vi "MainHost.vi"() -> ()   [LabVIEW 2014]
panel:
  out "XY ActivePath":cluster{dbl[], dbl[]}(graph)
  out "e 2":dbl
  out "y2 2":dbl
  out "x2 2":dbl
  out "y1 2":dbl
  out "x1 2":dbl
  out "pathActive":string
  out "dpActive":string
  out "Heading":dbl
  out "Pos x":dbl
  out "Pos y":dbl
  in  "isHIL":bool
  out "alpha Saturated":bool
  out "u Saturated":bool
  out "u":dbl[](array[numeric])
  out "alpha":dbl[](array[numeric])
  out "?":picture
  out "Vessel position":cluster{"x":dbl[], "y":dbl[]}[](graph)
  in  "TabModes":T1(tab)
  in  "u thruster 1":dbl(slide) min=-1.0 max=1.0 scale=-1.0..1.0
  in  "alpha 1":dbl(knob) min=-114.0 max=114.0 scale=-114.0..114.0
  in  "u thruster 2":dbl(slide) min=-1.0 max=1.0 scale=-1.0..1.0
  in  "alpha 2":dbl(knob) min=-114.0 max=114.0 scale=-114.0..114.0
  in  "u thruster 0":dbl(slide) min=-1.0 max=1.0 scale=-1.0..1.0
  in  "alpha 0":dbl(knob) min=-114.0 max=114.0 scale=-114.0..114.0
  in  "Switch to dashboard control thrus":bool
  in  "Switch to dashboard control force":bool
  in  "N force":dbl step=0.1
  in  "Y force":dbl step=0.2
  in  "X force":dbl step=0.2
  out "Reference initialization completed":bool
  in  "PID gains psi":T2={"proportional gain (Kc)"=0.5, "integral time (Ti, min)"=0.0, "derivative time (Td, min)"=0.0}
  in  "PID gains y":T2={"proportional gain (Kc)"=0.5, "integral time (Ti, min)"=0.0, "derivative time (Td, min)"=0.0}
  in  "PID gains x":T2={"proportional gain (Kc)"=0.5, "integral time (Ti, min)"=0.0, "derivative time (Td, min)"=0.0}
  in  "psi dp":dbl
  in  "y dp":dbl
  in  "x dp":dbl
  in  "Activate DP":bool
  in  "TabPaths":enum32{"Straight line", "Ellipse", "Waypoints"}(tab)
  in  "u_r":dbl step=0.1
  in  "PID gains u straight":T2={"proportional gain (Kc)"=0.5, "integral time (Ti, min)"=0.0, "derivative time (Td, min)"=0.0}
  in  "Ok straight":bool
  in  "Clear straight":bool
  out "XY straight":cluster{"X":dbl, "Y":dbl}[](graph)
  in  "Preview ellipse":bool
  in  "e":dbl
  in  "y2":dbl
  in  "x2":dbl
  in  "y1":dbl
  in  "x1":dbl
  in  "Ok ellipse":bool
  in  "Clear ellipse":bool
  out "XY ellipse":cluster{"x":dbl[], "y":dbl[]}(graph)
  in  "Activate DP Mode":bool
  in  "Ok wp":bool
  in  "Clear wp":bool
  out "XY Waypoints":cluster{"X":dbl, "Y":dbl}[](graph)
  in  "stop":bool
  # "Starting procedure: Choose setpoint, gains and activate DP. \nThe vessel will respond when the reference model has finished initializing."
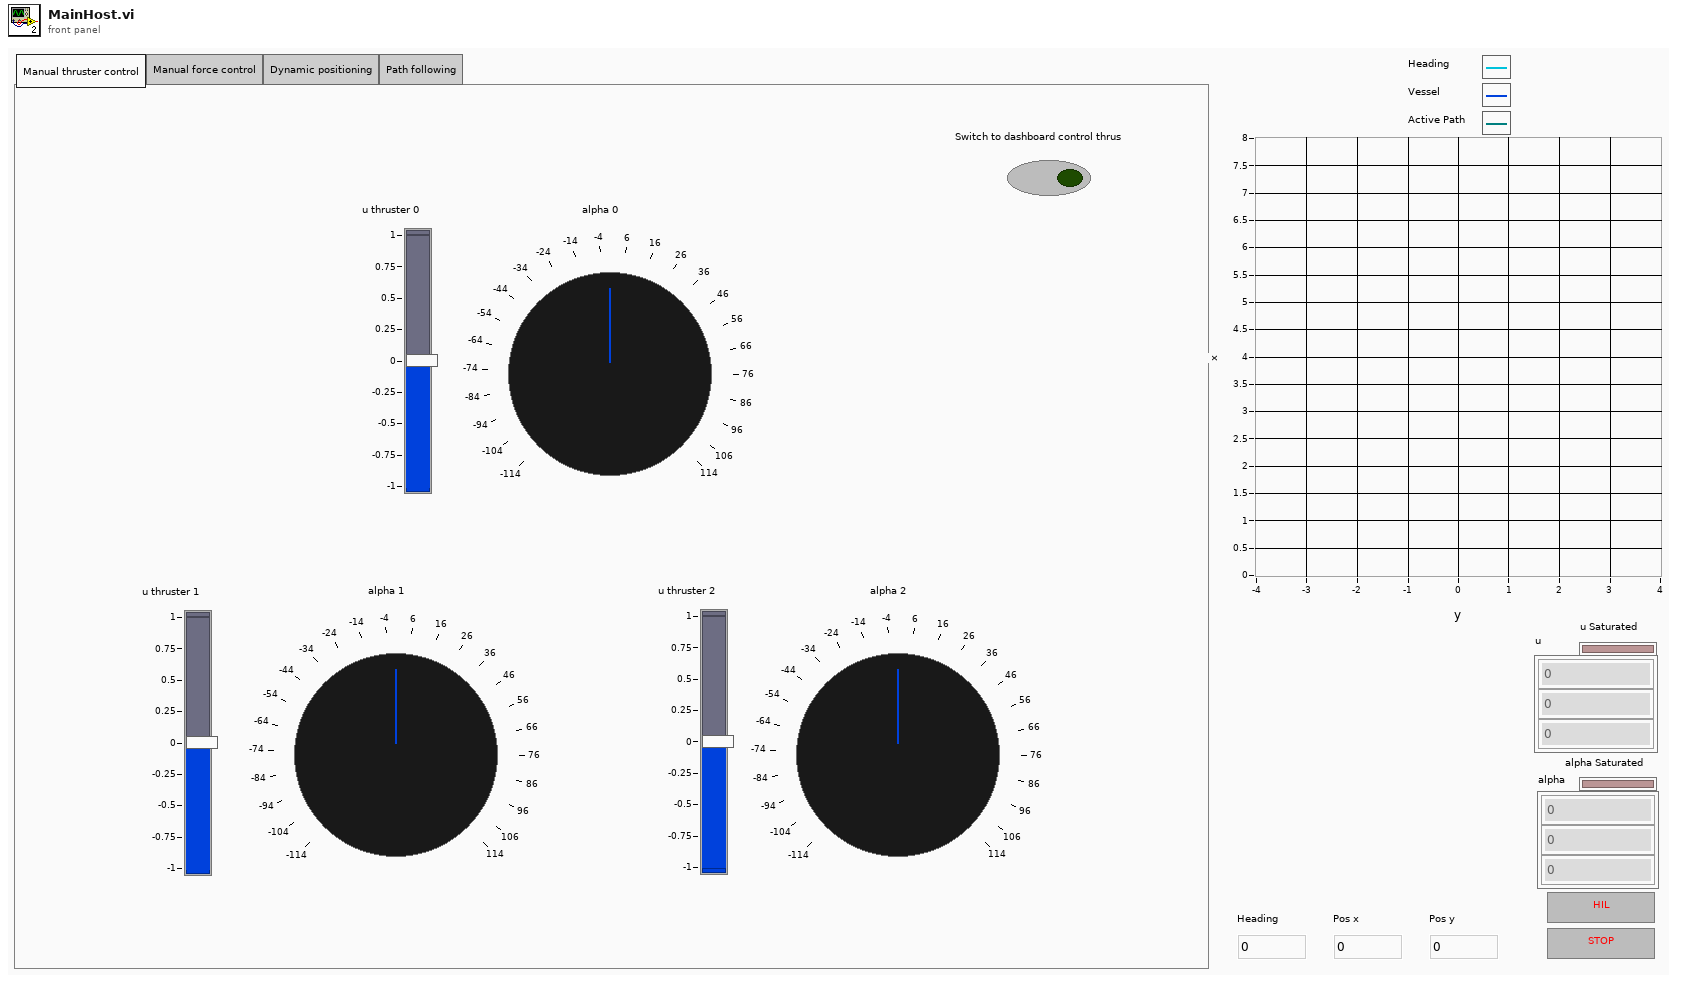
[diagram p1: front panel]
types:
  T1 = enum32{"Manual thruster control", "Manual force control", "Dynamic positioning", "Path following"}
  T2 = cluster{"proportional gain (Kc)":dbl, "integral time (Ti, min)":dbl, "derivative time (Td, min)":dbl}
  T3 = typedef "LVPoint32TypeDef.ctl" = cluster{"Horizontal":i32, "Vertical":i32}
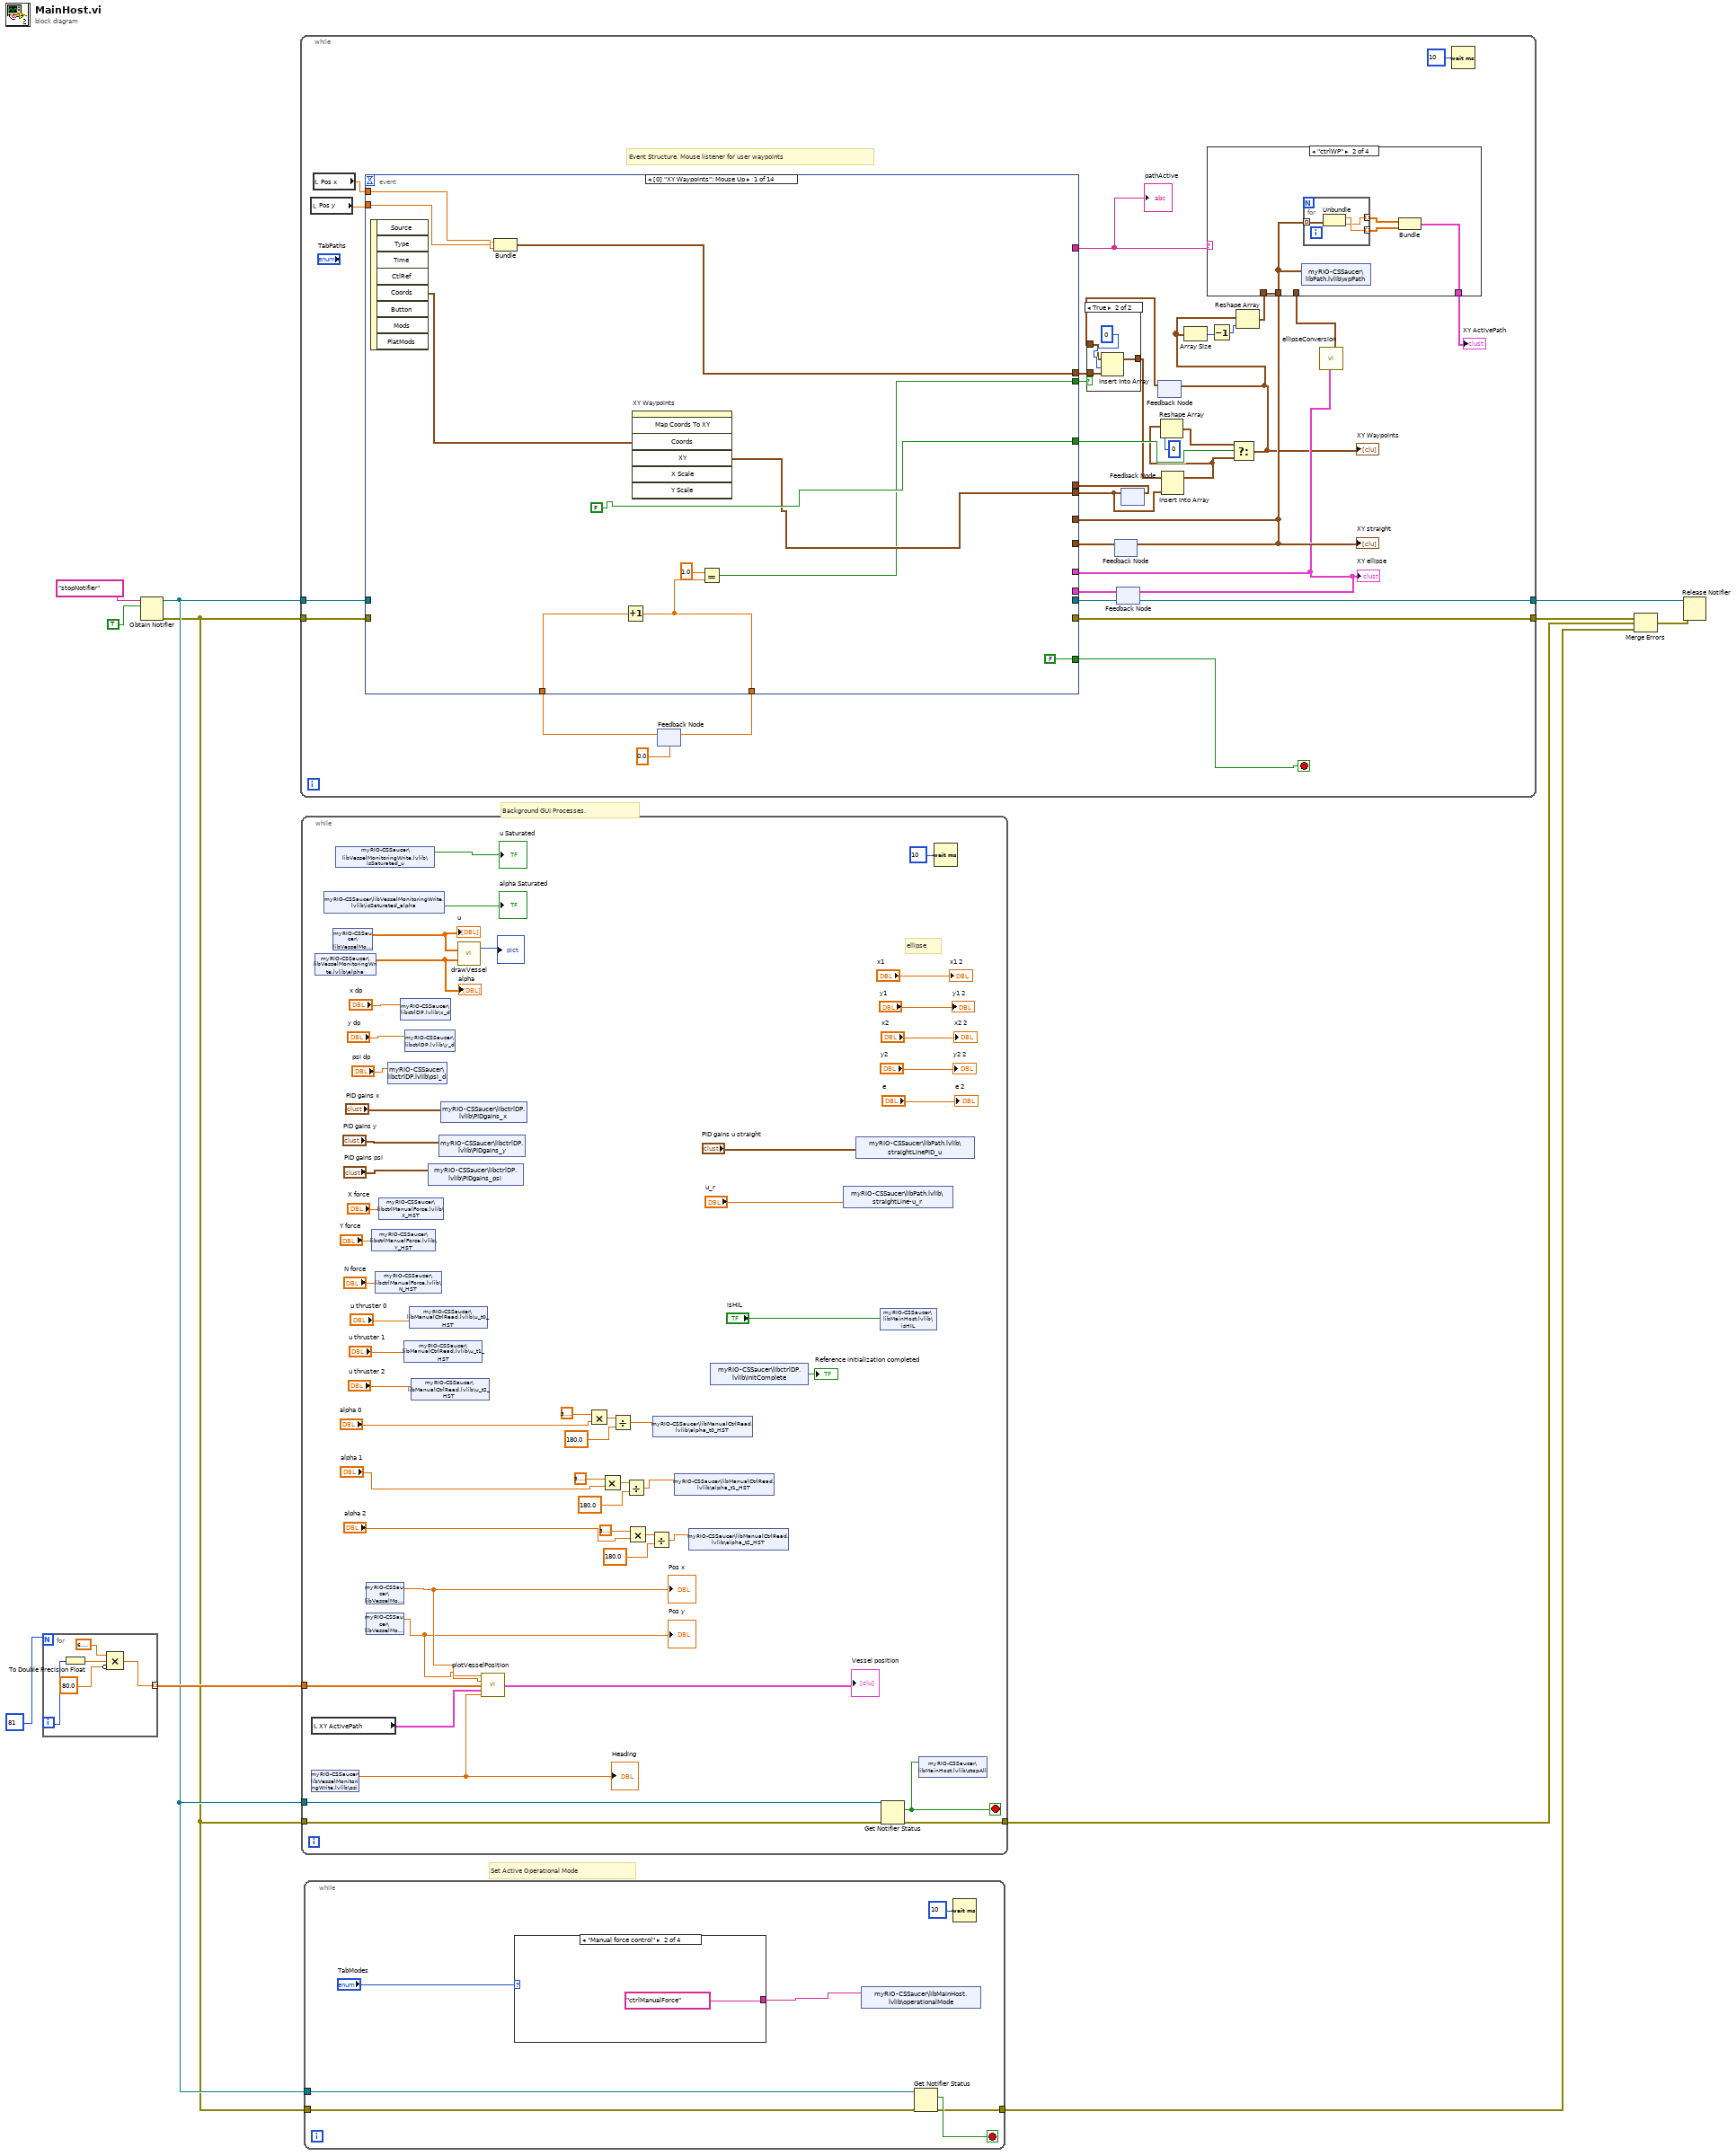
[diagram p0: block diagram]
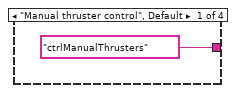
[diagram p2: hidden frame]
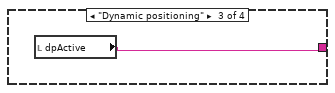
[diagram p3: hidden frame]
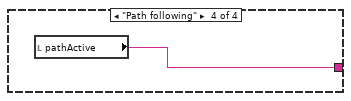
[diagram p4: hidden frame]
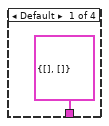
[diagram p6: hidden frame]
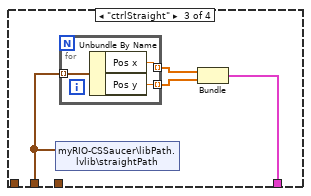
[diagram p7: hidden frame]
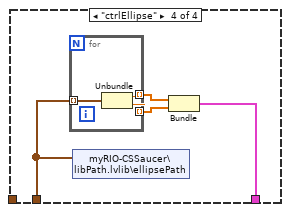
[diagram p8: hidden frame]
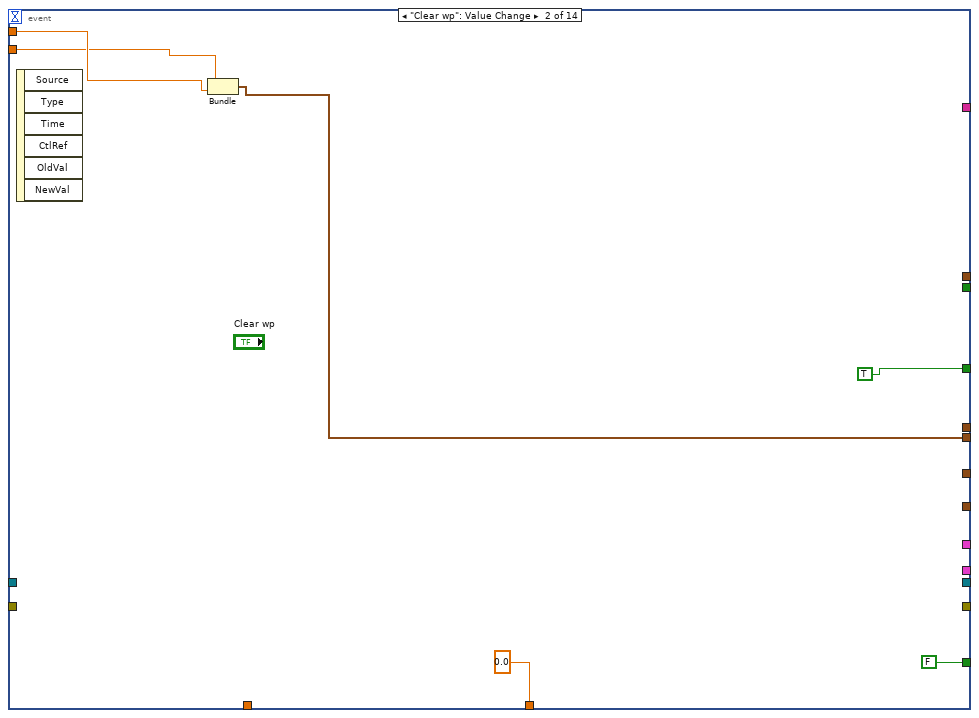
[diagram p9: hidden frame]
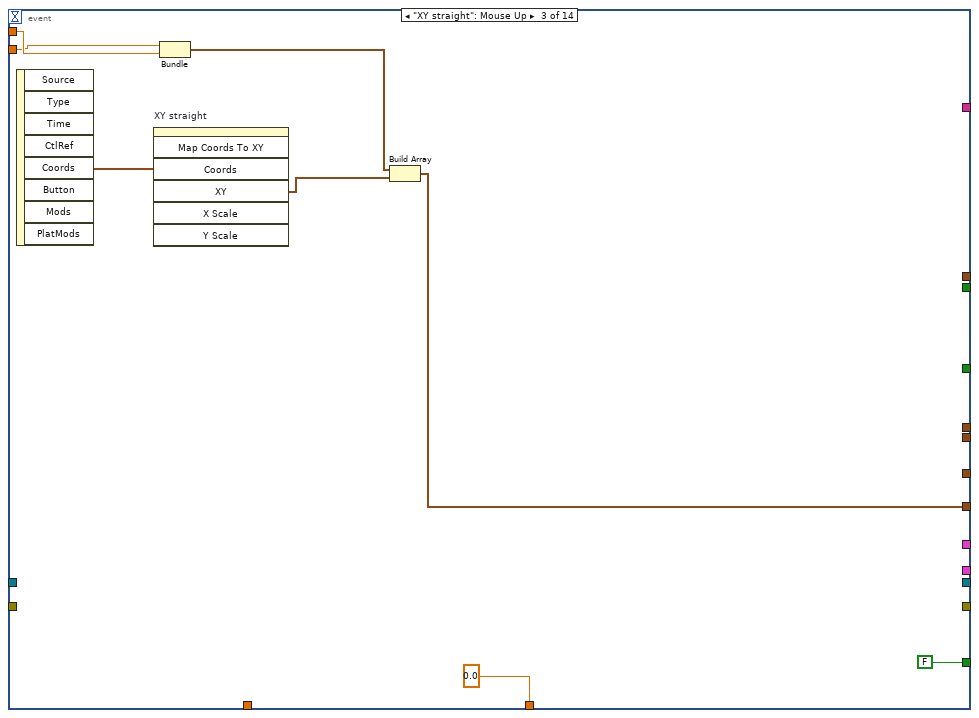
[diagram p10: hidden frame]
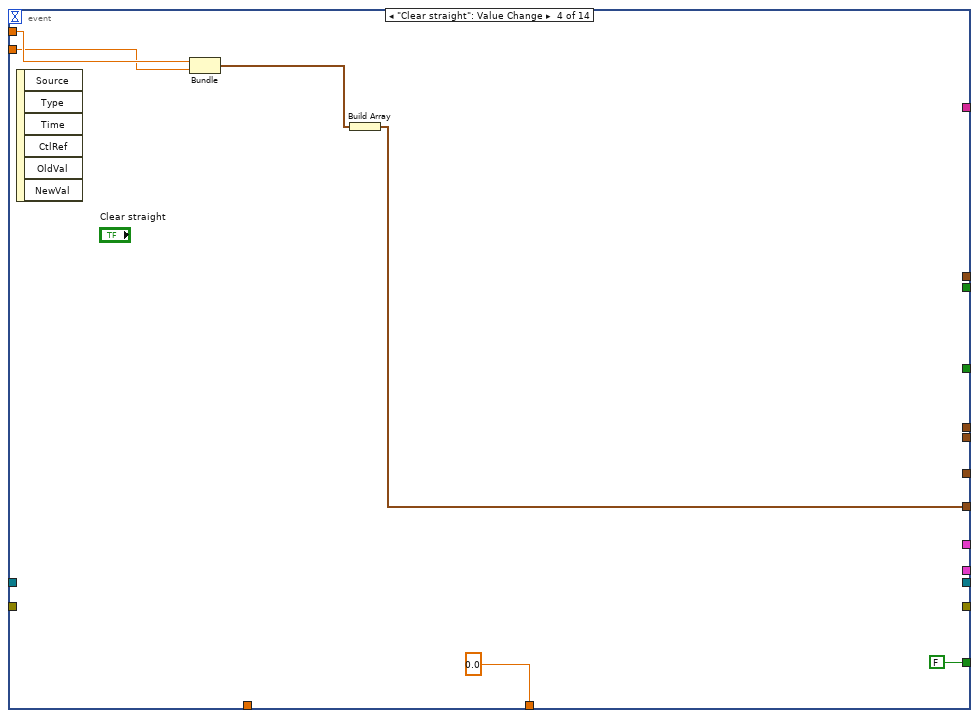
[diagram p11: hidden frame]
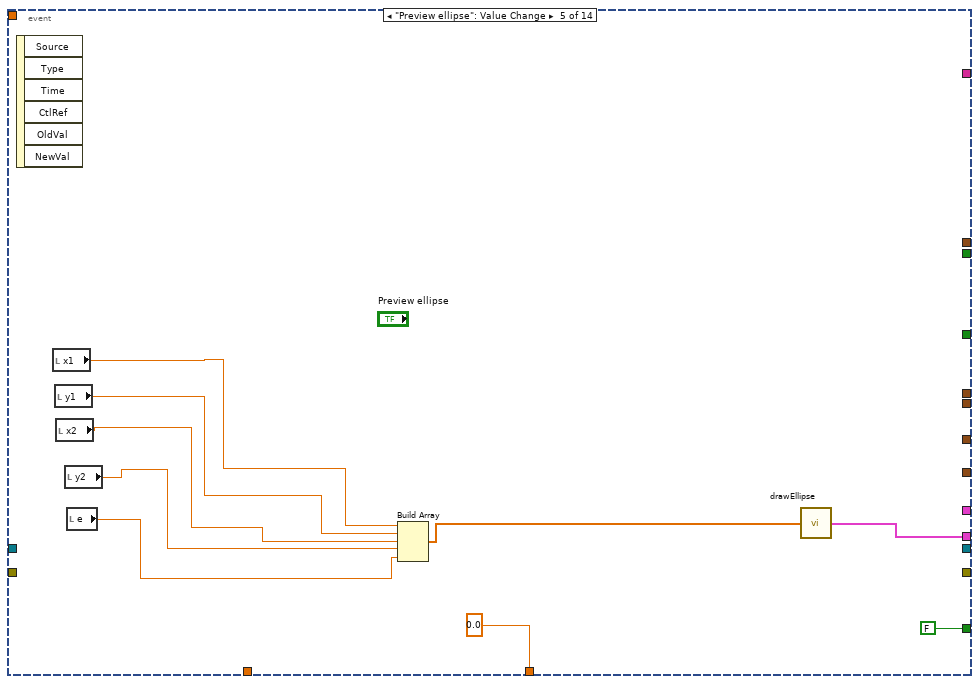
[diagram p12: hidden frame]
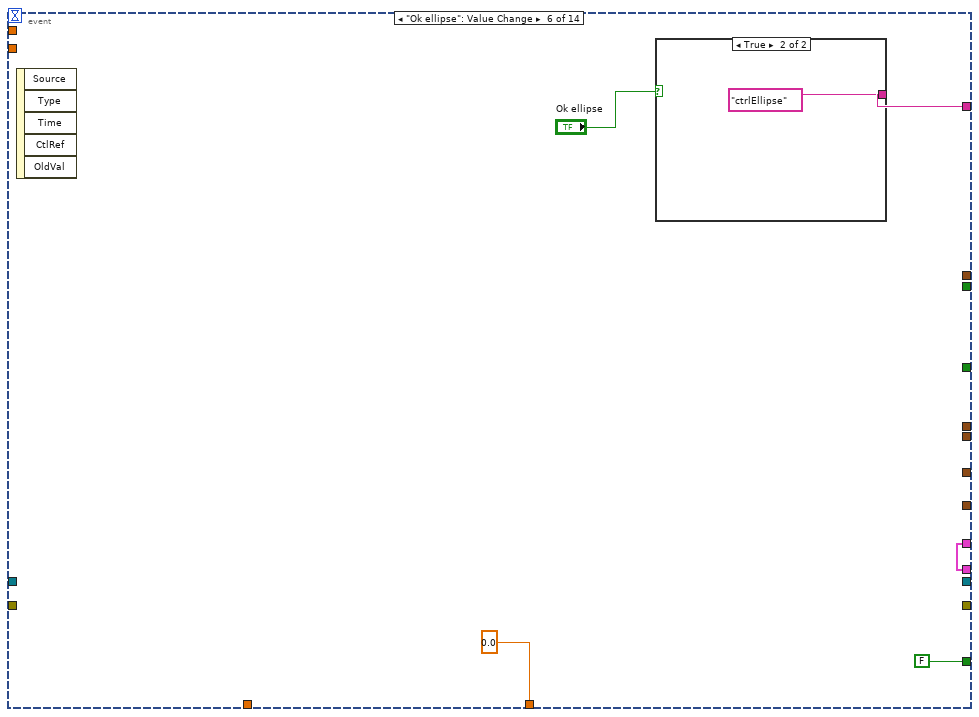
[diagram p13: hidden frame]
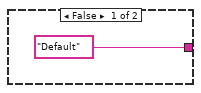
[diagram p14: hidden frame]
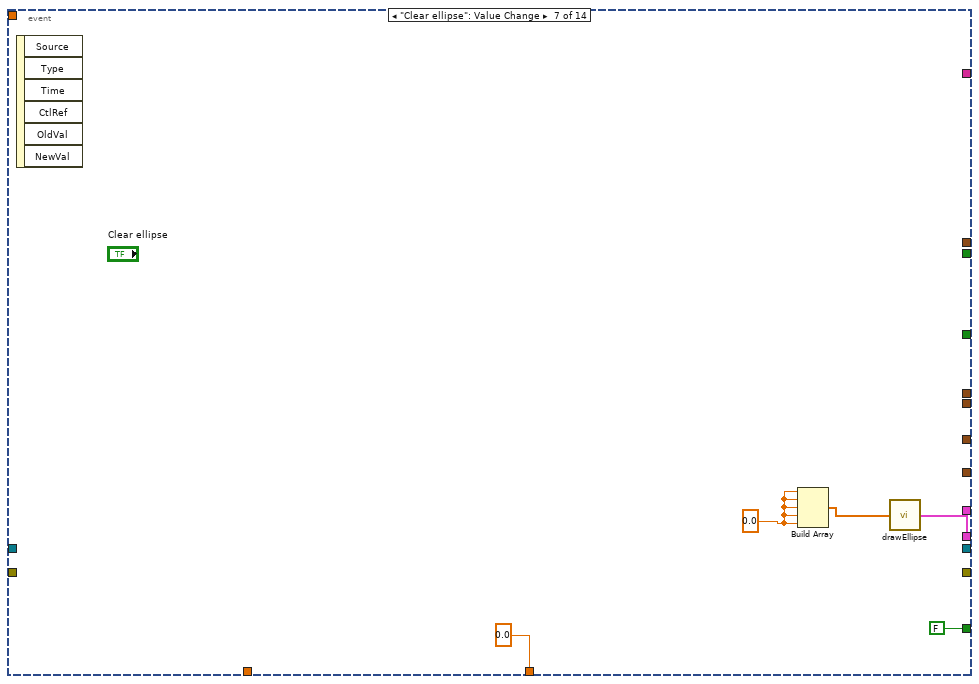
[diagram p15: hidden frame]
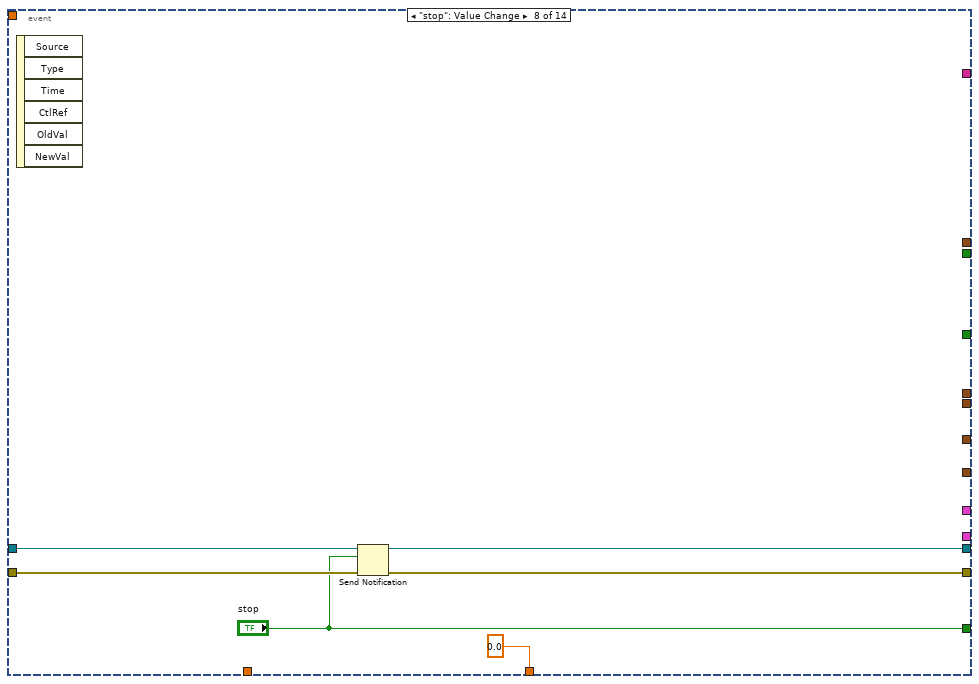
[diagram p16: hidden frame]
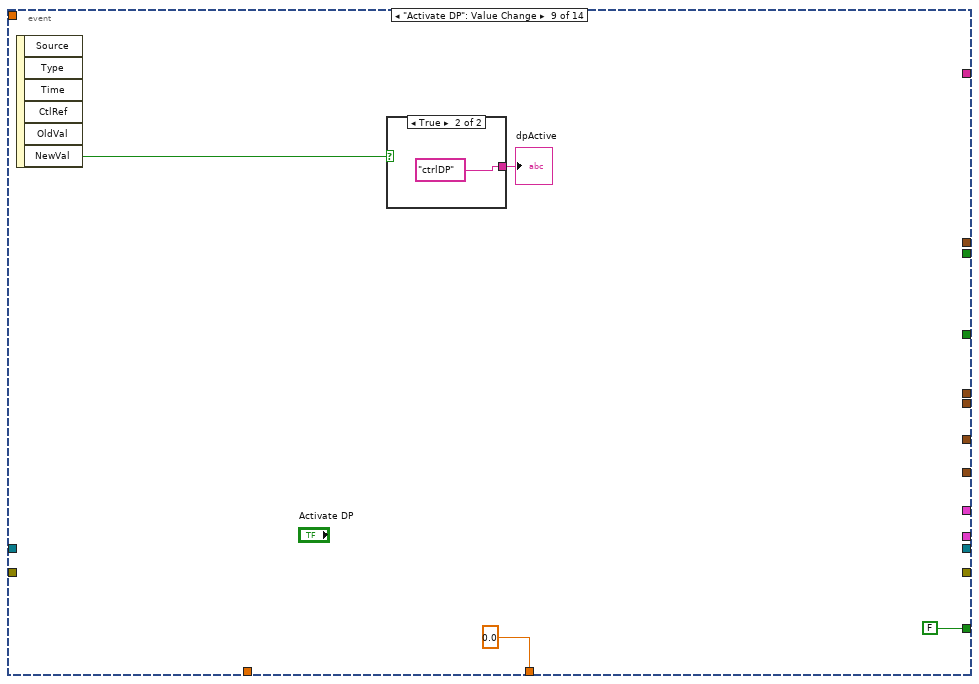
[diagram p17: hidden frame]
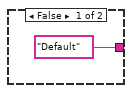
[diagram p18: hidden frame]
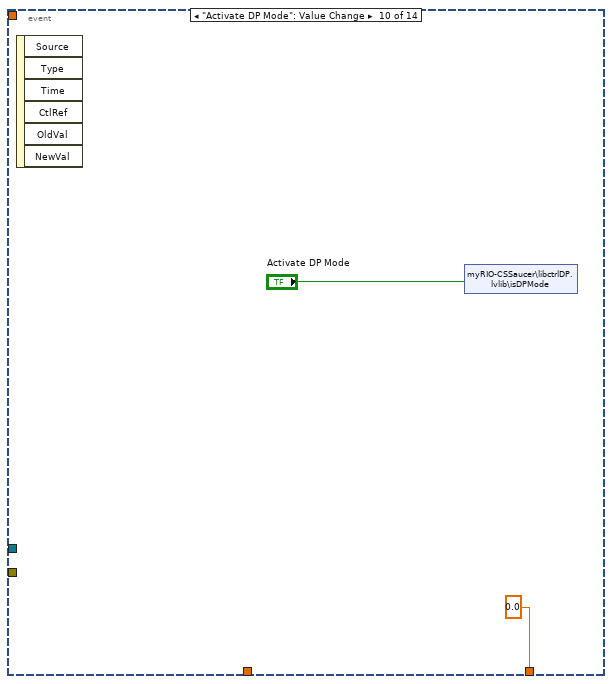
[diagram p19: hidden frame]
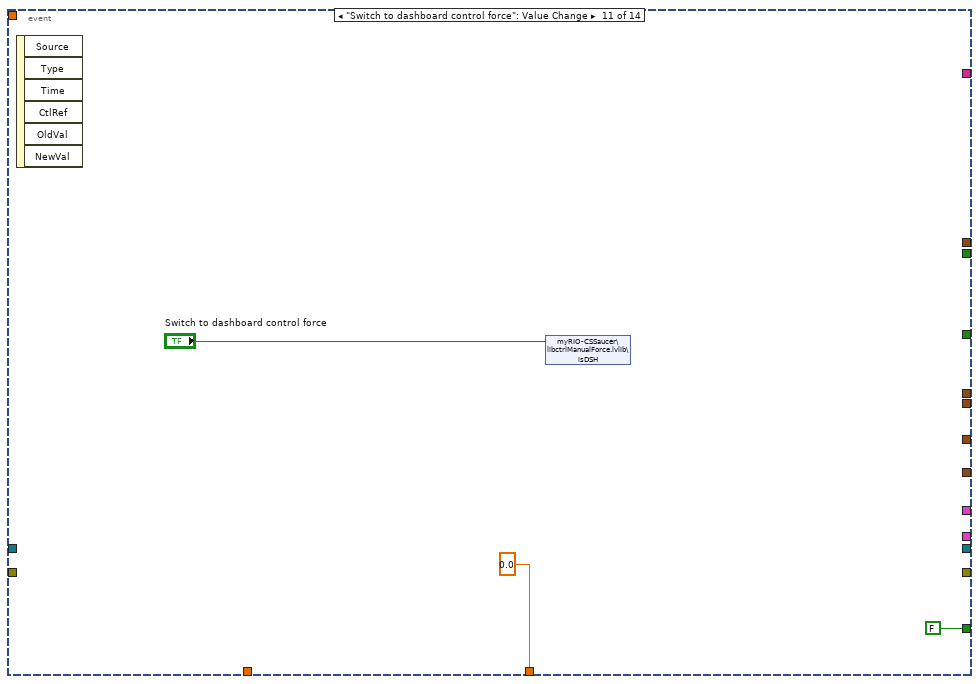
[diagram p20: hidden frame]
diagram:
  # "Background GUI Processes."
  # "Set Active Operational Mode"
  n1 = for {
    N: 81 -> [_]
    tunnel: [w12] -> w4 mode=indexing
    i -> [w14]
    n2 = To Double Precision Float(number=w14) -> (double precision float=w13:dbl)
    n3 = Compound Arithmetic op=MULTIPLY(6.283185307179586, w13, invert 80.0 ("value")) -> (w12:dbl)
  }
  n4 = Obtain Notifier(name (unnamed)="stopNotifier", notification data type=TRUE) -> (notifier out=w3:refnum<notifier>, error out=w2:errorcluster)  [unwired: 2 in, 1 out]
  n5 = while {
    tunnel: w3 -> [w43]
    tunnel: w2 -> [w42]
    tunnel: [w41] -> w7
    tunnel: [w40] -> w6
    stop <- w37 stop-if-true
    # "Event Structure. Mouse listener for user waypoints"
    n6 = local read "Pos y"() -> (w38:dbl)
    n7 = local read "Pos x"() -> (w39:dbl)
    n8 = feedback #1(0.0) -> (w21:dbl)
    n9 = feedback #2() -> (w34:cluster{"Pos x":dbl, "Pos y":dbl}[])  [unwired: 1 in]
    "XY straight" <- w34
    n10 = feedback #3() -> (w28:cluster{"x":dbl[], "y":dbl[]})  [unwired: 1 in]
    "XY ellipse" <- w28
    n11 = feedback #4() -> (w32:cluster{"Pos y":dbl, "Pos x":dbl})  [unwired: 1 in]
    n12 = event shown="[0] \"XY Waypoints\": Mouse Up" {
      selector: _ -> [_ _ _ _ _ _ _ _ _ _ _ _ _ _]
      dyn-events: _ -> [_ _ _ _ _ _ _ _ _ _ _ _ _ _]
      timeout: _ -> [_ _ _ _ _ _ _ _ _ _ _ _ _ _]
      tunnel: w38 -> [w76 w87 w93 w105 _ _ _ _ _ _ _ _ _ _]
      tunnel: w39 -> [w77 w88 w94 w106 _ _ _ _ _ _ _ _ _ _]
      tunnel: [_ _ w97 w103 _ _ _ _ _ _ _ _ w150 _] -> w35
      tunnel: [w84 w91 _ _ _ _ _ _ _ _ _ _ _ w155] -> w31
      tunnel: [FALSE TRUE _ _ _ _ _ _ _ _ _ _ _ _] -> w45
      tunnel: w43 -> [_ _ _ _ _ _ _ w133 _ _ _ _ _ _]
      tunnel: [_ _ _ _ _ _ _ w132 _ _ _ _ _ _] -> w41
      tunnel: w42 -> [_ _ _ _ _ _ _ w131 _ _ _ _ _ _]
      tunnel: [_ _ _ _ _ _ _ w130 _ _ _ _ _ _] -> w40
      tunnel: [FALSE FALSE FALSE FALSE FALSE FALSE FALSE "stop" FALSE _ FALSE FALSE FALSE FALSE] -> w37
      tunnel: [_ _ _ _ _ w120 _ _ _ _ _ _ w152 w158] -> w36
      tunnel: [_ _ _ _ w109 w118 w125 _ _ _ _ _ _ _] -> w33
      tunnel: w34 -> [_ _ _ _ _ _ _ _ _ _ _ _ w150 _]
      tunnel: w28 -> [_ _ _ _ _ w118 _ _ _ _ _ _ _ _]
      tunnel: w32 -> [_ _ _ _ _ _ _ _ _ _ _ _ _ w155]
      tunnel: w21 -> [w82 _ _ _ _ _ _ _ _ _ _ _ _ _]
      tunnel: [w81 0.0 0.0 0.0 0.0 0.0 0.0 0.0 0.0 0.0 0.0 0.0 0.0 _] -> w23
      tunnel: [w79 _ _ _ _ _ _ _ _ _ _ _ _ _] -> w18
      tunnel: [w78 _ _ _ _ _ _ _ _ _ _ _ _ _] -> w17
      event "XY Waypoints": Mouse Up {
        n13 = event-data() -> ("Coords"=w86:T3)  [unwired: 1 in, 7 out]
        n14 = Bundle("Pos y"=w76, "Pos x"=w77) -> (w79:cluster{"Pos y":dbl, "Pos x":dbl})  [unwired: 1 in]
        n15 = Increment(x=w82) -> (x+1=w81:dbl)
        n16 = invoke on="XY Waypoints" class="XYGraph (strict)" method="Map Coords To XY"("Coords"=w86) -> ("XY"=w84:cluster{"X":dbl, "Y":dbl})  [unwired: 6 in, 6 out]
        n17 = Equal?(x=1.0, y=w81) -> (x = y?=w78:bool)
      }
      event "Clear wp": Value Change {
        n18 = event-data() -> ()  [unwired: 1 in, 6 out]
        n19 = Bundle("Pos y"=w87, "Pos x"=w88) -> (w91:cluster{"Pos y":dbl, "Pos x":dbl})  [unwired: 1 in]
      }
      event "XY straight": Mouse Up {
        n20 = event-data() -> ("Coords"=w100:T3)  [unwired: 1 in, 7 out]
        n21 = invoke on="XY straight" class="XYGraph (strict)" method="Map Coords To XY"("Coords"=w100) -> ("XY"=w98:cluster{"X":dbl, "Y":dbl})  [unwired: 6 in, 6 out]
        n22 = Bundle("Pos y"=w93, "Pos x"=w94) -> (w99:cluster{"Pos y":dbl, "Pos x":dbl})  [unwired: 1 in]
        n23 = Build Array(w99, w98) -> (w97:cluster{"X":dbl, "Y":dbl}[])
      }
      event "Clear straight": Value Change {
        n24 = event-data() -> ()  [unwired: 1 in, 6 out]
        n25 = Bundle("Pos x"=w106, "Pos y"=w105) -> (w104:cluster{"Pos x":dbl, "Pos y":dbl})  [unwired: 1 in]
        n26 = Build Array(w104) -> (w103:cluster{"Pos x":dbl, "Pos y":dbl}[])
      }
      event "Preview ellipse": Value Change {
        n27 = event-data() -> ()  [unwired: 1 in, 6 out]
        n28 = local read "x1"() -> (w115:dbl)
        n29 = local read "y1"() -> (w114:dbl)
        n30 = local read "x2"() -> (w113:dbl)
        n31 = local read "y2"() -> (w112:dbl)
        n32 = local read "e"() -> (w111:dbl)
        n33 = Build Array(w115, w114, w113, w112, w111) -> (w110:dbl[])
        n34 = call "drawEllipse.vi"("ellipse in"=w110) -> ("XY ellipse"=w109:cluster{"x":dbl[], "y":dbl[]})  [unwired: 4 in]
      }
      event "Ok ellipse": Value Change {
        n35 = event-data() -> ()  [unwired: 1 in, 5 out]
        n36 = case shown="True" "Ok ellipse" {
          tunnel: ["Default" "ctrlEllipse"] -> w120
          frame False {
          }
          frame True {
          }
        }
      }
      event "Clear ellipse": Value Change {
        w127 = 0.0 ("element")
        n37 = event-data() -> ()  [unwired: 1 in, 6 out]
        n38 = Build Array(w127, w127, w127, w127, w127) -> (w126:dbl[])
        n39 = call "drawEllipse.vi"("ellipse in"=w126) -> ("XY ellipse"=w125:cluster{"x":dbl[], "y":dbl[]})  [unwired: 4 in]
      }
      event "stop": Value Change {
        n40 = event-data() -> ()  [unwired: 1 in, 6 out]
        n41 = Send Notification(notification="stop", notifier=w133, error in (no error)=w131) -> (notifier out=w132:refnum<notifier>, error out=w130:errorcluster)
      }
      event "Activate DP": Value Change {
        n42 = event-data() -> ("NewVal"=w137:bool)  [unwired: 1 in, 5 out]
        n43 = case shown="True" w137 {
          tunnel: ["Default" "ctrlDP"] -> w136
          frame False {
          }
          frame True {
          }
        }
        "dpActive" <- w136
      }
      event "Activate DP Mode": Value Change {
        n44 = event-data() -> ()  [unwired: 1 in, 6 out]
        n45 = shared-variable "myRIO-CSSaucer\\libctrlDP.lvlib\\isDPMode"("Activate DP Mode") -> ()  [unwired: 1 in, 1 out]
      }
      event "Switch to dashboard control force": Value Change {
        n46 = event-data() -> ()  [unwired: 1 in, 6 out]
        n47 = shared-variable "myRIO-CSSaucer\\libctrlManualForce.lvlib\\isDSH"("Switch to dashboard control force") -> ()  [unwired: 1 in, 1 out]
      }
      event "Switch to dashboard control thrus": Value Change {
        n48 = event-data() -> ()  [unwired: 1 in, 6 out]
        n49 = shared-variable "myRIO-CSSaucer\\libManualCtrlRead.lvlib\\isDashboardActive"("Switch to dashboard control thrus") -> ()  [unwired: 1 in, 1 out]
      }
      event "Ok straight": Value Change {
        n50 = event-data() -> ()  [unwired: 1 in, 6 out]
        n51 = case shown="True" "Ok straight" {
          tunnel: ["Default" "ctrlStraight"] -> w152
          frame False {
          }
          frame True {
          }
        }
      }
      event "Ok wp": Value Change {
        n52 = event-data() -> ()  [unwired: 1 in, 6 out]
        n53 = case shown="True" "Ok wp" {
          tunnel: ["Default" "ctrlWP"] -> w158
          frame False {
          }
          frame True {
          }
        }
      }
    }
    "pathActive" <- w36
    n54 = feedback-in #1(w23) -> ()
    n55 = feedback-in #2(w35) -> ()
    n56 = feedback-in #3(w33) -> ()
    n57 = feedback-in #4(w31) -> ()
    n58 = feedback #5() -> (w19:cluster{"Pos y":dbl, "Pos x":dbl}[])  [unwired: 1 in]
    n59 = case shown="True" w17 {
      tunnel: [w49 w50] -> w20
      tunnel: w19 -> [w49 w52]
      tunnel: w18 -> [_ w51]
      frame False {
      }
      frame True {
        n60 = Insert Into Array(array=w52, index=0, new element=w51) -> (w50:cluster{"Pos y":dbl, "Pos x":dbl}[])
      }
    }
    n61 = Insert Into Array(array=w20, new element=w31) -> (w44:cluster{"Pos y":dbl, "Pos x":dbl}[])  [unwired: 1 in]
    n62 = Reshape Array(w44, 0 ("dimension size")) -> (w47:cluster{"Pos y":dbl, "Pos x":dbl}[])
    n63 = Select(t=w47, s=w45, f=w44) -> (s? t:f=w26:cluster{"Pos y":dbl, "Pos x":dbl}[])
    "XY Waypoints" <- w26
    n64 = feedback-in #5(w26) -> ()
    n65 = Array Size(array=w26) -> (size(s)=w27:i32)
    n66 = Decrement(x=w27) -> (x-1=w25:i32)
    n67 = Reshape Array(w26, w25) -> (w24:cluster{"Pos y":dbl, "Pos x":dbl}[])
    n68 = call "ellipseConversion.vi"("XY ellipse 2"=w28) -> ("Array"=w30:cluster{dbl, dbl}[])  [unwired: 10 in]
    n69 = case shown="\"ctrlWP\"" w36 {
      tunnel: w34 -> [_ _ w65 _]
      tunnel: w24 -> [_ w58 _ _]
      tunnel: w30 -> [_ _ _ w72]
      tunnel: [cluster{dbl[], dbl[]} {[], []} w57 w64 w71] -> w29
      frame Default {
      }
      frame "ctrlWP" {
        n70 = shared-variable "myRIO-CSSaucer\\libPath.lvlib\\wpPath"(w58) -> ()  [unwired: 1 in, 1 out]
        n71 = for {
          tunnel: w58 -> [w61] mode=indexing
          tunnel: [w59] -> w56 mode=indexing
          tunnel: [w60] -> w55 mode=indexing
          n72 = Unbundle(w61) -> ("Pos y"=w60:dbl, "Pos x"=w59:dbl)
        }
        n73 = Bundle(w56, w55) -> (w57:cluster{dbl[], dbl[]})  [unwired: 1 in]
      }
      frame "ctrlStraight" {
        n74 = shared-variable "myRIO-CSSaucer\\libPath.lvlib\\straightPath"(w65) -> ()  [unwired: 1 in, 1 out]
        n75 = for {
          tunnel: w65 -> [w68] mode=indexing
          tunnel: [w67] -> w63 mode=indexing
          tunnel: [w66] -> w62 mode=indexing
          n76 = Unbundle By Name(w68) -> ("Pos x"=w67:dbl, "Pos y"=w66:dbl)
        }
        n77 = Bundle(w63, w62) -> (w64:cluster{dbl[], dbl[]})  [unwired: 1 in]
      }
      frame "ctrlEllipse" {
        n78 = for {
          tunnel: w72 -> [w75] mode=indexing
          tunnel: [w74] -> w69 mode=indexing
          tunnel: [w73] -> w70 mode=indexing
          n79 = Unbundle(w75) -> (w74:dbl, w73:dbl)
        }
        n80 = shared-variable "myRIO-CSSaucer\\libPath.lvlib\\ellipsePath"(w72) -> ()  [unwired: 1 in, 1 out]
        n81 = Bundle(w69, w70) -> (w71:cluster{dbl[], dbl[]})  [unwired: 1 in]
      }
    }
    "XY ActivePath" <- w29
    n82 = Wait (ms)(milliseconds to wait=u32 10) -> ()  [unwired: 1 out]
  }
  n83 = while {
    tunnel: w3 -> [w207]
    tunnel: w2 -> [w206]
    tunnel: [w205] -> w8
    tunnel: w4 -> [w168]
    stop <- w165 stop-if-true
    # "ellipse"
    n84 = local read "XY ActivePath"() -> (w167:cluster{dbl[], dbl[]})
    n85 = shared-variable "myRIO-CSSaucer\\libVesselMonitoringWrite.lvlib\\psi"() -> (w169:dbl)  [unwired: 1 in, 1 out]
    "Heading" <- w169
    n86 = shared-variable "myRIO-CSSaucer\\libVesselMonitoringWrite.lvlib\\alpha"() -> (w209:dbl[])  [unwired: 1 in, 1 out]
    "alpha" <- w209
    n87 = shared-variable "myRIO-CSSaucer\\libVesselMonitoringWrite.lvlib\\isSaturated_alpha"() -> (→"alpha Saturated":bool)  [unwired: 1 in, 1 out]
    n88 = shared-variable "myRIO-CSSaucer\\libVesselMonitoringWrite.lvlib\\u"() -> (w208:dbl[])  [unwired: 1 in, 1 out]
    "u" <- w208
    n89 = shared-variable "myRIO-CSSaucer\\libVesselMonitoringWrite.lvlib\\isSaturated_u"() -> (→"u Saturated":bool)  [unwired: 1 in, 1 out]
    n90 = shared-variable "myRIO-CSSaucer\\libVesselMonitoringWrite.lvlib\\x"() -> (w162:dbl)  [unwired: 1 in, 1 out]
    "Pos x" <- w162
    n91 = shared-variable "myRIO-CSSaucer\\libVesselMonitoringWrite.lvlib\\y"() -> (w161:dbl)  [unwired: 1 in, 1 out]
    "Pos y" <- w161
    n92 = shared-variable "myRIO-CSSaucer\\libctrlManualForce.lvlib\\Y_HST"("Y force") -> ()  [unwired: 1 in, 1 out]
    n93 = shared-variable "myRIO-CSSaucer\\libctrlManualForce.lvlib\\N_HST"("N force") -> ()  [unwired: 1 in, 1 out]
    n94 = shared-variable "myRIO-CSSaucer\\libctrlManualForce.lvlib\\X_HST"("X force") -> ()  [unwired: 1 in, 1 out]
    n95 = shared-variable "myRIO-CSSaucer\\libctrlDP.lvlib\\psi_d"("psi dp") -> ()  [unwired: 1 in, 1 out]
    n96 = shared-variable "myRIO-CSSaucer\\libctrlDP.lvlib\\x_d"("x dp") -> ()  [unwired: 1 in, 1 out]
    n97 = shared-variable "myRIO-CSSaucer\\libManualCtrlRead.lvlib\\u_t1_HST"("u thruster 1") -> ()  [unwired: 1 in, 1 out]
    n98 = shared-variable "myRIO-CSSaucer\\libctrlDP.lvlib\\y_d"("y dp") -> ()  [unwired: 1 in, 1 out]
    n99 = shared-variable "myRIO-CSSaucer\\libManualCtrlRead.lvlib\\u_t0_HST"("u thruster 0") -> ()  [unwired: 1 in, 1 out]
    n100 = shared-variable "myRIO-CSSaucer\\libManualCtrlRead.lvlib\\u_t2_HST"("u thruster 2") -> ()  [unwired: 1 in, 1 out]
    n101 = shared-variable "myRIO-CSSaucer\\libctrlDP.lvlib\\PIDgains_psi"("PID gains psi") -> ()  [unwired: 1 in, 1 out]
    n102 = shared-variable "myRIO-CSSaucer\\libctrlDP.lvlib\\PIDgains_y"("PID gains y") -> ()  [unwired: 1 in, 1 out]
    n103 = shared-variable "myRIO-CSSaucer\\libctrlDP.lvlib\\PIDgains_x"("PID gains x") -> ()  [unwired: 1 in, 1 out]
    n104 = call "drawVessel.vi"("alpha"=w209, "u"=w208) -> (1:→"?":picture)  [unwired: 1 in]
    n105 = call "plotVesselPosition.vi"("x"=w161, "y"=w162, "angles"=w168, "Cluster"=w167, "psi"=w169) -> ("XY Graph"=→"Vessel position":cluster{"x":dbl[], "y":dbl[]}[])  [unwired: 10 in]
    n106 = Multiply(x=3.141592653589793, y="alpha 0") -> (x*y=w191:dbl)
    n107 = Multiply(x=3.141592653589793, y="alpha 1") -> (x*y=w188:dbl)
    n108 = Divide(x=w191, y=180.0) -> (x/y=w181:dbl)
    n109 = Divide(x=w188, y=180.0) -> (x/y=w180:dbl)
    n110 = Multiply(x=3.141592653589793, y="alpha 2") -> (x*y=w185:dbl)
    n111 = Divide(x=w185, y=180.0) -> (x/y=w179:dbl)
    n112 = shared-variable "myRIO-CSSaucer\\libManualCtrlRead.lvlib\\alpha_t0_HST"(w181) -> ()  [unwired: 1 in, 1 out]
    n113 = shared-variable "myRIO-CSSaucer\\libManualCtrlRead.lvlib\\alpha_t1_HST"(w180) -> ()  [unwired: 1 in, 1 out]
    n114 = shared-variable "myRIO-CSSaucer\\libManualCtrlRead.lvlib\\alpha_t2_HST"(w179) -> ()  [unwired: 1 in, 1 out]
    n115 = shared-variable "myRIO-CSSaucer\\libctrlDP.lvlib\\initComplete"() -> (→"Reference initialization completed":bool)  [unwired: 1 in, 1 out]
    n116 = shared-variable "myRIO-CSSaucer\\libPath.lvlib\\straightLine-u_r"("u_r") -> ()  [unwired: 1 in, 1 out]
    n117 = shared-variable "myRIO-CSSaucer\\libPath.lvlib\\straightLinePID_u"("PID gains u straight") -> ()  [unwired: 1 in, 1 out]
    n118 = shared-variable "myRIO-CSSaucer\\libMainHost.lvlib\\isHIL"("isHIL") -> ()  [unwired: 1 in, 1 out]
    n119 = Get Notifier Status(notifier=w207, error in (no error)=w206) -> (current notification=w165:bool, error out=w205:errorcluster)  [unwired: 3 out]
    n120 = shared-variable "myRIO-CSSaucer\\libMainHost.lvlib\\stopAll"(w165) -> ()  [unwired: 1 in, 1 out]
    n121 = Wait (ms)(milliseconds to wait=u32 10) -> ()  [unwired: 1 out]
    "x1 2" <- "x1"
    "y1 2" <- "y1"
    "x2 2" <- "x2"
    "y2 2" <- "y2"
    "e 2" <- "e"
  }
  n122 = while {
    tunnel: w3 -> [w217]
    tunnel: w2 -> [w216]
    tunnel: [w215] -> w1
    stop <- w218 stop-if-true
    n123 = case shown="\"Manual force control\"" "TabModes" {
      tunnel: ["ctrlManualThrusters" "ctrlManualForce" w222 w223] -> w213
      frame "Manual thruster control", Default {
      }
      frame "Manual force control" {
      }
      frame "Dynamic positioning" {
        n124 = local read "dpActive"() -> (w222:string)
      }
      frame "Path following" {
        n125 = local read "pathActive"() -> (w223:string)
      }
    }
    n126 = shared-variable "myRIO-CSSaucer\\libMainHost.lvlib\\operationalMode"(w213) -> ()  [unwired: 1 in, 1 out]
    n127 = Get Notifier Status(notifier=w217, error in (no error)=w216) -> (current notification=w218:bool, error out=w215:errorcluster)  [unwired: 3 out]
    n128 = Wait (ms)(milliseconds to wait=u32 10) -> ()  [unwired: 1 out]
  }
  n129 = Merge Errors(w6, w8, w1) -> (w5:errorcluster)
  n130 = Release Notifier(notifier=w7, error in (no error)=w5) -> ()  [unwired: 1 in, 3 out]
